vi "Rotation2D_Get Inverse.vi"(11 "ROTATION":T1 {"SIN" format="%13.4f"; "COS" format="%13.4f"; "VALUE" format="%13.4f"}) -> (3 "Inverse ROTATION":T1 {"SIN" format="%13.4f"; "COS" format="%13.4f"; "VALUE" format="%13.4f"})   [LabVIEW 2020, in "Swerve_Odometry_SEN.lvlib"]
doc: "Takes the inverse of the current rotation. This is simply the negative of the current angular value.\n\nParameters:\n - IN ROTATION - This ROTATION data structure\n\nResults:\n - OUT ROTATION - The negated ROTATION data structure."
uses:
  Swerve_Odometry_SEN.lvlib
  Cluster_ROTATION2D.ctl
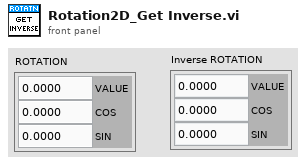
[diagram p1: front panel]
types:
  T1 = typedef "Swerve_Odometry_SEN.lvlib/Cluster_ROTATION2D.ctl" = cluster{"VALUE":dbl, "COS":dbl, "SIN":dbl}
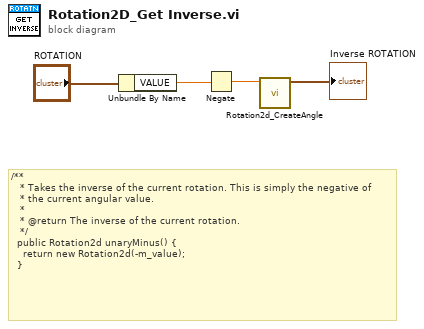
[diagram p0: block diagram]
diagram:
  # "/**\n   * Takes the inverse of the current rotation. This is simply the negative of\n   * the current angular value.\n   *\n   * @return The inverse of the current rotation.\n   */\n  public Rotation2d unaryMinus() {\n    return new Rotation2d(-m_value);\n  }"
  n1 = Unbundle By Name("ROTATION") -> ("VALUE"=w3:dbl)
  n2 = Negate(x=w3) -> (-x=w2:dbl)
  n3 = call "Rotation2d_CreateAngle.vi"("Angle (Radians)"=w2) -> ("ROTATION"=→"Inverse ROTATION":T1)  [unwired: 10 in]
